vi "Addres string (SubVI).vi"(11 "Адрес":i32) -> (3 "String":string)   [LabVIEW 2017, in "LV_Unicorn.lvlib"]
uses:
  LV_Unicorn.lvlib
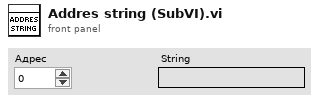
[diagram p1: front panel]
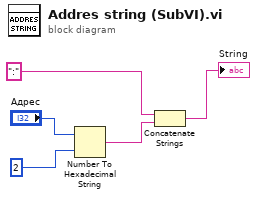
[diagram p0: block diagram]
diagram:
  n1 = Number To Hexadecimal String(1:i16 2 ("width (-)"), 2:"Адрес") -> (0:w1:string)
  n2 = Concatenate Strings(":" ("string"), w1) -> (→"String":string)
